vi "CreateFolder.vi"(11 "appended path":path) -> (2 "file or folder exists?":bool, 3 "dup path":path)   [LabVIEW 2018, in "File IO.lvlib"]
uses:
  File IO.lvlib
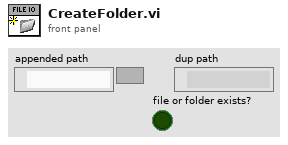
[diagram p1: front panel]
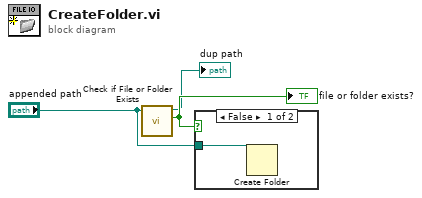
[diagram p0: block diagram]
diagram:
  n1 = call <vilib>:"Check if File or Folder Exists.vi"("path"="appended path") -> ("file or folder exists?"=w3:bool, "dup path"=→"dup path":path)  [unwired: 8 in, 1 out]
  "file or folder exists?" <- w3
  n2 = case shown="False" w3 {
    tunnel: "appended path" -> [w4 _]
    frame False {
      n3 = Create Folder(path (use dialog)=w4) -> ()  [unwired: 2 in, 3 out]
    }
    frame True {
      # "Folder exists"
    }
  }
